vi "Max Search.vi"() -> ()   [LabVIEW 2019]
panel:
  out "Max":dbl
  out "Iterations":i32
  in  "Number of Iterations":i32
  out "Random Number":dbl
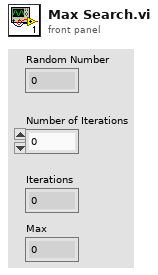
[diagram p1: front panel]
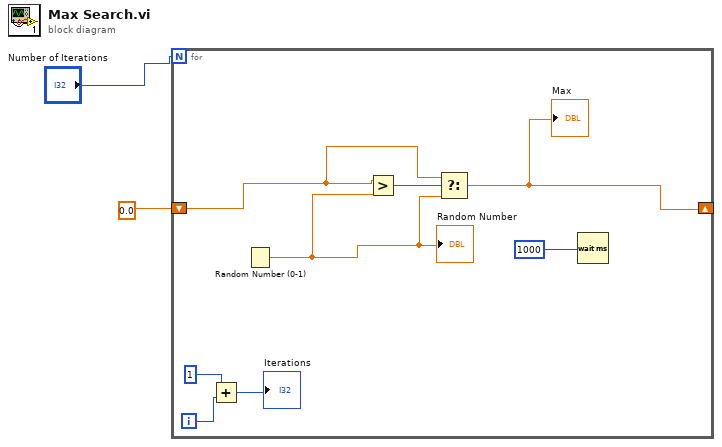
[diagram p0: block diagram]
diagram:
  n1 = for {
    N: "Number of Iterations" -> [_]
    shift-right: [w8] -> _
    shift-left: 0.0 -> [w7]
    i -> [w4]
    n2 = Add(x=1, y=w4) -> (x+y=→"Iterations":i32)
    n3 = Random Number (0-1)() -> (number: 0 to 1=w6:dbl)
    "Random Number" <- w6
    n4 = Greater?(x=w7, y=w6) -> (0:w9:bool)
    n5 = Select(t=w7, s=w9, f=w6) -> (s? t:f=w8:dbl)
    "Max" <- w8
    n6 = Wait (ms)(milliseconds to wait=u32 1000) -> ()  [unwired: 1 out]
  }
